vi "Select Channel.vi"(10 "AO Channel":T2, 11 "Data":T1) -> (3 "Analog Output":refnum<class "niInstr Instruction Framework Context v1 Host.lvclass">)   [LabVIEW 2017, in "Test Bench.lvlib"]
uses:
  Test Bench.lvlib
  AO Channels.ctl
  Scan Engine Variables.ctl
  <instrlib>/_niInstr/FIFO Register Bus/v1/Host/niInstr FIFO Register Bus v1 Host.lvclass
  <instrlib>/_niInstr/Instruction Framework/v1/Host/Instruction Framework Context/niInstr Instruction Framework Context v1 Host.lvclass
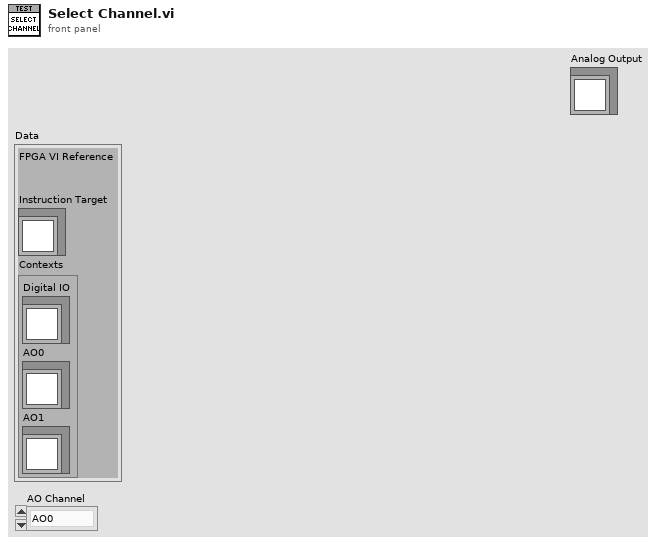
[diagram p1: front panel]
types:
  T1 = typedef "Test Bench.lvlib/Scan Engine Variables.ctl" = cluster{"FPGA VI Reference":refnum<k20>, "Instruction Target":refnum<class "niInstr FIFO Register Bus v1 Host.lvclass">, "Contexts":cluster{"Digital IO":refnum<class "niInstr Instruction Framework Context v1 Host.lvclass">, "AO0":refnum<class "niInstr Instruction Framework Context v1 Host.lvclass">, "AO1":refnum<class "niInstr Instruction Framework Context v1 Host.lvclass">}}
  T2 = typedef "Test Bench.lvlib/AO Channels.ctl" = enum16{"AO0", "AO1"}
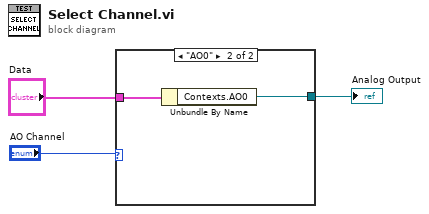
[diagram p0: block diagram]
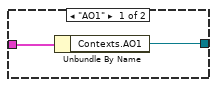
[diagram p2: hidden frame]
diagram:
  n1 = case shown="\"AO0\"" "AO Channel" {
    tunnel: "Data" -> [w5 w7]
    tunnel: [w4 w6] -> w1
    frame "AO1" {
      n2 = Unbundle By Name(w5) -> ("Contexts.AO1"=w4:refnum<class "niInstr Instruction Framework Context v1 Host.lvclass">)
    }
    frame "AO0" {
      n3 = Unbundle By Name(w7) -> ("Contexts.AO0"=w6:refnum<class "niInstr Instruction Framework Context v1 Host.lvclass">)
    }
  }
  "Analog Output" <- w1
